vi "SMC Heater= Message.vi"(0 "Switch Heater":bool) -> ()   [LabVIEW 2010]
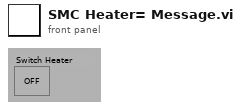
[diagram p1: front panel]
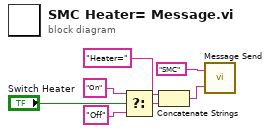
[diagram p0: block diagram]
diagram:
  n1 = Select(t="On" ("Message"), s="Switch Heater", f="Off" ("Message")) -> (s? t:f=w4:string)
  n2 = Concatenate Strings("Heater=" ("Message"), w4) -> (w3:string)
  n3 = call "Message Send.vi"("Message"=w3, "Destination"="SMC" ("Destination(s)")) -> ()
